vi "SetVoltage.vi"(3 "Voltage":dbl, 4 "error in":errorcluster, 5 "connection ID":refnum<k5>) -> (0 "False":bool, 1 "error out":errorcluster, 2 "connection ID out":refnum<k5>)   [LabVIEW 2013]
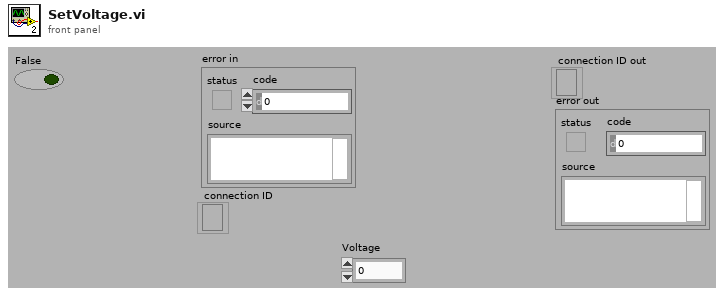
[diagram p1: front panel]
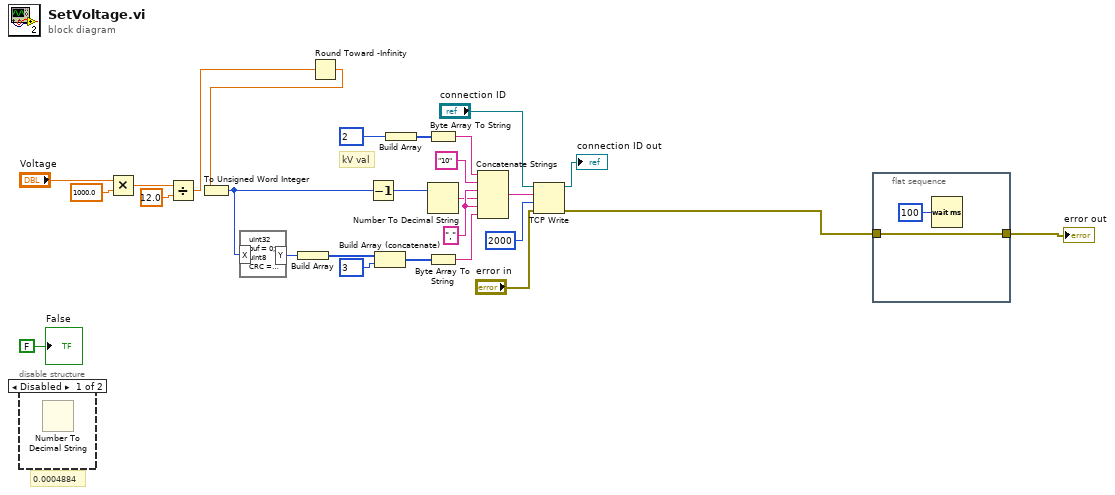
[diagram p0: block diagram]
diagram:
  w16 = "," ("string")
  # "kV val"
  # "0.0004884"
  n1 = disable-structure shown="Disabled" {
    frame Disabled {
      n2 = Number To Decimal String() -> ()  [unwired: 1 in, 2 out]
    }
    frame Enabled {
    }
  }
  n3 = Multiply(x="Voltage", y=1000.0) -> (x*y=w6:dbl)
  n4 = Divide(x=w6, y=12.0) -> (x/y=w4:dbl)
  n5 = Round Toward -Infinity(1:w4) -> (0:w3:dbl)
  n6 = To Unsigned Word Integer(number=w3) -> (unsigned 16bit integer=w10:u16)
  n7 = formula code="uInt32 buf = 0;\nuInt8 CRC = 0;\nuInt8 Y = 0;\n\nbuf = 0x31 + 0x30  + X + 0x2C;\nbuf = ~ buf;\nbuf = buf & 0x000000FF;\nCRC = buf;\nCRC &= 0x7F;\nCRC |= 0x40;\nCRC++;\nY = CRC;"("X"=w10) -> ("Y"=w14:u8)
  n8 = Build Array(w14) -> (w13:u8[])
  n9 = Decrement(x=w10) -> (x-1=w5:u16)
  n10 = Build Array (concatenate)(w13, u8 3 ("y")) -> (w21:u8[])
  n11 = Build Array(u8 2 ("y")) -> (w19:u8[])
  n12 = Byte Array To String(unsigned byte array=w19) -> (string=w18:string)
  n13 = Number To Decimal String(number=w5) -> (decimal integer string=w9:string)  [unwired: 1 in]
  n14 = Byte Array To String(unsigned byte array=w21) -> (string=w12:string)
  n15 = Concatenate Strings(w18, "10" ("string"), w16, w9, w16, w12) -> (w15:string)
  n16 = TCP Write(connection ID="connection ID", data in=w15, error in (no error)="error in", 9:2000 ("timeout ms (25000)")) -> (connection ID out=→"connection ID out":refnum<k5>, error out=w1:errorcluster)  [unwired: 1 out]
  n17 = flat-sequence {
    tunnel: [w29] -> w2
    tunnel: w1 -> [w29]
    frame #0 {
      n18 = Wait (ms)(milliseconds to wait=u32 100) -> ()  [unwired: 1 out]
    }
  }
  "error out" <- w2
  "False" <- FALSE
